vi "qp_quadratic objective function.vi"(2 "c":dbl[](array[numeric]), 3 "X":dbl[](array[numeric]), 4 "NI":i32, 5 "Q":dbl[][](array[numeric])) -> (1 "ob":dbl)   [LabVIEW 2018, in "NI_Gmath.lvlib"]
uses:
  NI_Gmath.lvlib
  Real Dot Product.vi
  A x Vector.vi
  NI_AALBase.lvlib
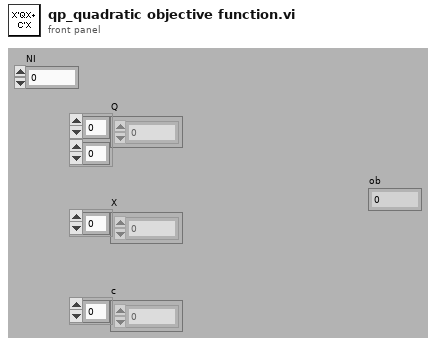
[diagram p1: front panel]
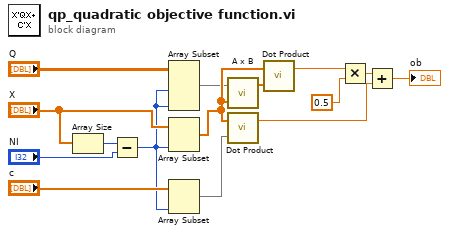
[diagram p0: block diagram]
diagram:
  n1 = Array Size(array="X") -> (size(s)=w8:i32)
  n2 = Subtract(x=w8, y="NI") -> (x-y=w1:i32)
  n3 = Array Subset(array="Q", length (row)=w1, length (col)=w1) -> (w4:dbl[][])  [unwired: 2 in]
  n4 = Array Subset(array="X", length=w1) -> (w6:dbl[])  [unwired: 1 in]
  n5 = Array Subset(array="c", length=w1) -> (w2:dbl[])  [unwired: 1 in]
  n6 = call-poly "A x B.vi"("Vector"=w6, "A"=w4) -> ("A x Vector"=w15:dbl[])  [unwired: 1 out]
  n7 = call-poly "Dot Product.vi"("Y Vector"=w2, "X Vector"=w6) -> ("X * Y"=w11:dbl)  [unwired: 1 out]
  n8 = call-poly "Dot Product.vi"("Y Vector"=w15, "X Vector"=w6) -> ("X * Y"=w14:dbl)  [unwired: 1 out]
  n9 = Multiply(x=w14, y=0.5) -> (x*y=w12:dbl)
  n10 = Add(x=w12, y=w11) -> (x+y=→"ob":dbl)
